vi "Refresh Systems.vi"() -> (3 "Systems":string[](array[string]))   [LabVIEW 2016]
uses:
  <vilib>/Message/Open (Sync).vi
  <vilib>/Message/Subscribe (Sync).vi
  <vilib>/Message/Publish (Sync).vi
  <vilib>/Message/Unsubscribe (Sync).vi
  <vilib>/Message/Close (Sync).vi
  <vilib>/Message/Message.lvlib
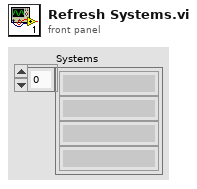
[diagram p1: front panel]
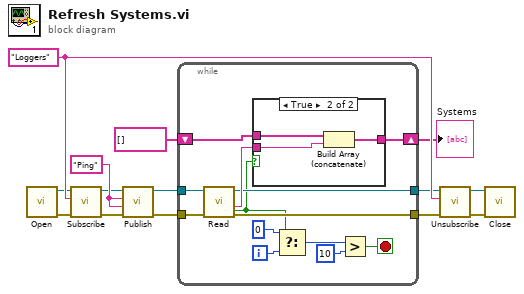
[diagram p0: block diagram]
diagram:
  w5 = "Ping" ("topic")
  w14 = "Loggers" ("topic")
  n1 = call-poly <vilib>:"Open.vi"() -> ("error out"=w3:errorcluster, "message sync reference"=w4:refnum<k21>)  [unwired: 10 in]
  n2 = call-poly <vilib>:"Subscribe.vi"("error in (no error)"=w3, "topic"=w14, "message sync reference in"=w4) -> ("error out"=w1:errorcluster, "message sync reference out"=w2:refnum<k21>)  [unwired: 7 in]
  n3 = call-poly <vilib>:"Publish.vi"("error in (no error)"=w1, "message"=w5, "topic"=w5, "message sync reference in"=w2) -> ("error out"=w7:errorcluster, "message sync reference out"=w6:refnum<k21>)  [unwired: 6 in]
  n4 = while {
    tunnel: w6 -> [w27]
    tunnel: w7 -> [w26]
    shift-right: [w19] -> w9
    shift-left: string[] [] -> [w18]
    tunnel: [w17] -> w12
    tunnel: [w16] -> w13
    i -> [w25]
    stop <- w22 stop-if-true
    n5 = call <vilib>:"Read.vi"("error in (no error)"=w26, "message sync reference in"=w27) -> ("error out"=w17:errorcluster, "message"=w20:string, "message sync reference out"=w16:refnum<k21>, "dequeueStatus"=w15:bool)  [unwired: 5 in, 1 out]
    n6 = case shown="True" w15 {
      tunnel: w20 -> [_ w30]
      tunnel: [w28 w29] -> w19
      tunnel: w18 -> [w28 w31]
      frame False {
      }
      frame True {
        n7 = Build Array (concatenate)(w31, w30) -> (w29:string[])
      }
    }
    n8 = Select(t=0, s=w15, f=w25) -> (s? t:f=w23:i32)
    n9 = Greater?(x=w23, y=10) -> (0:w22:bool)
  }
  "Systems" <- w9
  n10 = call-poly <vilib>:"Unsubscribe.vi"("error in (no error)"=w12, "topic"=w14, "message sync reference in"=w13) -> ("error out"=w10:errorcluster, "message sync referenc out"=w11:refnum<k21>)  [unwired: 7 in]
  n11 = call-poly <vilib>:"Close.vi"("error in"=w10, "message sync reference"=w11) -> ()  [unwired: 9 in, 1 out]
